vi "test-pose2d.vi"(8 "error in (no error)":errorcluster) -> (0 "error out":errorcluster, 3 "All PASSED":bool)   [LabVIEW 2019]
uses:
  <vilib>/Rock Robotics/WPI/ThirdParty/JAS_Junk/TrajLib/Translation_Equals.vi
  <vilib>/Rock Robotics/WPI/ThirdParty/JAS_Junk/TrajLib/Rotation_Equals.vi
  <vilib>/Rock Robotics/WPI/ThirdParty/JAS_Junk/TrajLib/Transform_Create_PosePose.vi
  <vilib>/Rock Robotics/WPI/ThirdParty/JAS_Junk/TrajLib/Pose_TransformBy.vi
  <vilib>/Rock Robotics/WPI/ThirdParty/JAS_Junk/TrajLib/Util_CalcDist.vi
  <vilib>/Rock Robotics/WPI/ThirdParty/JAS_Junk/TrajLib/Rotation_UnaryMinus.vi
  <vilib>/Rock Robotics/WPI/ThirdParty/JAS_Junk/TrajLib/Translation_RotateBy.vi
  <vilib>/Rock Robotics/WPI/ThirdParty/JAS_Junk/TrajLib/Translation_Minus.vi
  <vilib>/Rock Robotics/WPI/ThirdParty/JAS_Junk/TrajLib/Rotation_Minus.vi
  <vilib>/Rock Robotics/WPI/ThirdParty/JAS_Junk/TrajLib/Translation_Plus.vi
  <vilib>/Rock Robotics/WPI/ThirdParty/JAS_Junk/TrajLib/Rotation_Plus.vi
  <vilib>/Rock Robotics/WPI/ThirdParty/JAS_Junk/TrajLib/Rotation_RotateBy.vi
  <vilib>/Rock Robotics/WPI/ThirdParty/JAS_Junk/TrajLib/Rotation_CreateXY.vi
  <vilib>/Rock Robotics/WPI/ThirdParty/JAS_Junk/TrajLib/Trajectory_Library.lvlib
panel:
  out "T4 -- Deg -- 0":dbl
  out "T4 -- y -- 0":dbl
  out "T4 -- X -- 0":dbl
  out "T3 - False":bool
  out "T2 - True":bool
  out "T1 -- Deg -- 0":dbl
  out "T1 -- y -- 0":dbl
  out "T1 -- X -- 0":dbl
  out "T0 -- Deg -- 0":dbl
  out "T0 -- y -- 0":dbl
  out "T0 -- X -- 0":dbl
  # "Pose 2D test"
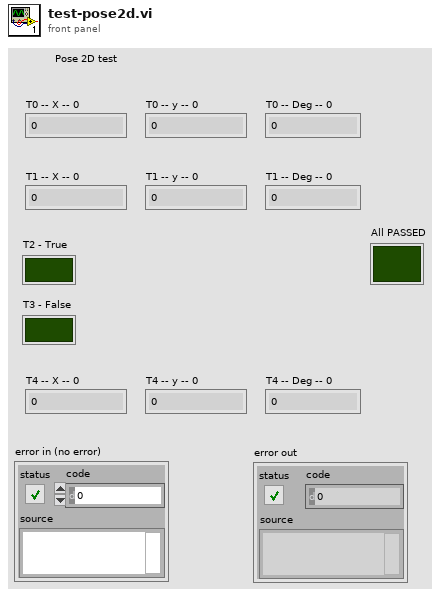
[diagram p1: front panel]
types:
  T1 = typedef "Trajectory_Library.lvlib/TRANSLATION2D.ctl" = cluster{"X":dbl, "Y":dbl}
  T2 = typedef "Trajectory_Library.lvlib/ROTATION2D.ctl" = cluster{"VALUE":dbl, "COS":dbl, "SIN":dbl}
  T3 = typedef "Trajectory_Library.lvlib/TRANSFORM2D.ctl" = cluster{"TRANSLATION":T1, "ROTATION":T2}
  T4 = typedef "Trajectory_Library.lvlib/POSE2D.ctl" = cluster{"TRANSLATION":T1, "ROTATION":T2}
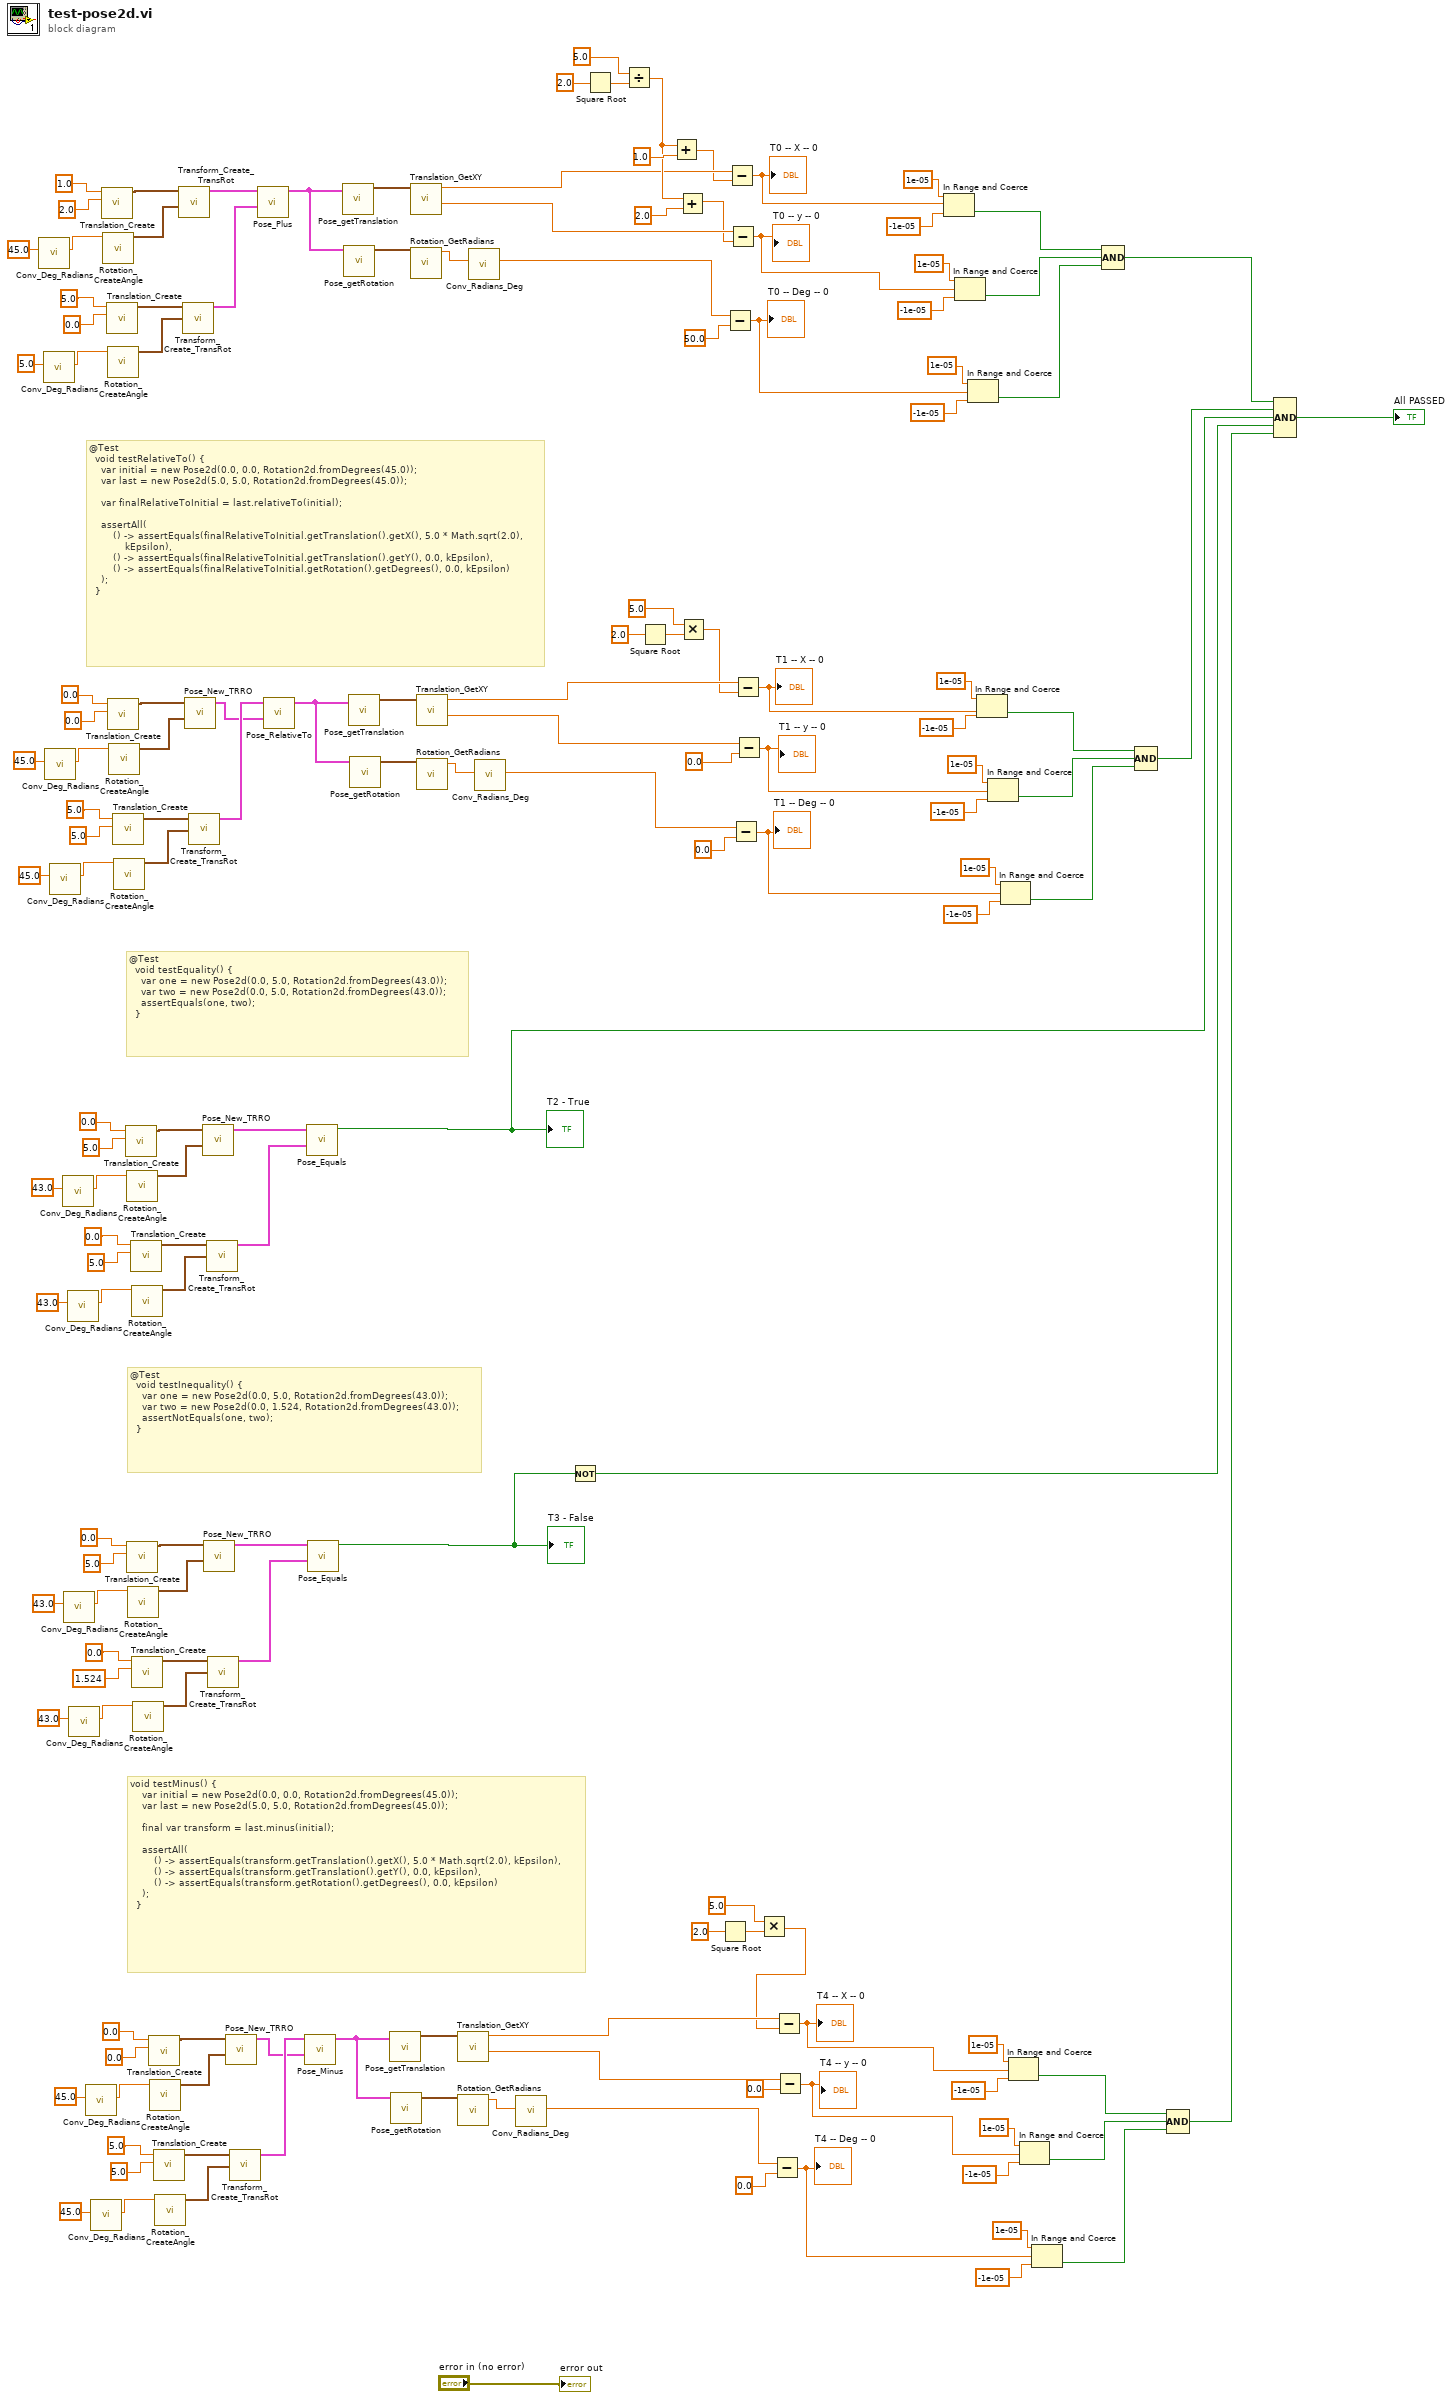
[diagram p0: block diagram]
diagram:
  # "void testMinus() {\n    var initial = new Pose2d(0.0, 0.0, Rotation2d.fromDegrees(45.0));\n    var last = new Pose2d(5.0, 5.0, Rotation2d.fromDegrees(45.0));\n\n    final var transform = last.minus(initial);\n\n    assertAll(\n        () -> assertEquals(transform.getTranslation().getX(), 5.0 * Math.sqrt(2.0), kEpsilon),\n        () -> assertEquals(transform.getTranslation().getY(), 0.0, kEpsilon),\n        () -> assertEquals(transform.getRotation().getDegrees(), 0.0, kEpsilon)\n    );\n  }"
  # "@Test\n  void testInequality() {\n    var one = new Pose2d(0.0, 5.0, Rotation2d.fromDegrees(43.0));\n    var two = new Pose2d(0.0, 1.524, Rotation2d.fromDegrees(43.0));\n    assertNotEquals(one, two);\n  }"
  # "@Test\n  void testEquality() {\n    var one = new Pose2d(0.0, 5.0, Rotation2d.fromDegrees(43.0));\n    var two = new Pose2d(0.0, 5.0, Rotation2d.fromDegrees(43.0));\n    assertEquals(one, two);\n  }"
  # "@Test\n  void testRelativeTo() {\n    var initial = new Pose2d(0.0, 0.0, Rotation2d.fromDegrees(45.0));\n    var last = new Pose2d(5.0, 5.0, Rotation2d.fromDegrees(45.0));\n\n    var finalRelativeToInitial = last.relativeTo(initial);\n\n    assertAll(\n        () -> assertEquals(finalRelativeToInitial.getTranslation().getX(), 5.0 * Math.sqrt(2.0),\n            kEpsilon),\n        () -> assertEquals(finalRelativeToInitial.getTranslation().getY(), 0.0, kEpsilon),\n        () -> assertEquals(finalRelativeToInitial.getRotation().getDegrees(), 0.0, kEpsilon)\n    );\n  }"
  n1 = call <vilib>:"Conv_Deg_Radians.vi"("Degress"=45.0) -> ("Radians"=w153:dbl)  [unwired: 10 in]
  n2 = call <vilib>:"Conv_Deg_Radians.vi"("Degress"=5.0) -> ("Radians"=w148:dbl)  [unwired: 10 in]
  n3 = call <vilib>:"Conv_Deg_Radians.vi"("Degress"=45.0) -> ("Radians"=w123:dbl)  [unwired: 10 in]
  n4 = call <vilib>:"Conv_Deg_Radians.vi"("Degress"=45.0) -> ("Radians"=w118:dbl)  [unwired: 10 in]
  n5 = call <vilib>:"Conv_Deg_Radians.vi"("Degress"=43.0) -> ("Radians"=w96:dbl)  [unwired: 10 in]
  n6 = call <vilib>:"Conv_Deg_Radians.vi"("Degress"=43.0) -> ("Radians"=w82:dbl)  [unwired: 10 in]
  n7 = call <vilib>:"Conv_Deg_Radians.vi"("Degress"=43.0) -> ("Radians"=w91:dbl)  [unwired: 10 in]
  n8 = call <vilib>:"Conv_Deg_Radians.vi"("Degress"=43.0) -> ("Radians"=w77:dbl)  [unwired: 10 in]
  n9 = call <vilib>:"Conv_Deg_Radians.vi"("Degress"=45.0) -> ("Radians"=w68:dbl)  [unwired: 10 in]
  n10 = call <vilib>:"Conv_Deg_Radians.vi"("Degress"=45.0) -> ("Radians"=w63:dbl)  [unwired: 10 in]
  n11 = call <vilib>:"Translation_Create.vi"("Y"=2.0, "X"=1.0) -> ("TRANSLATION"=w152:T1)  [unwired: 9 in]
  n12 = call <vilib>:"Rotation_CreateAngle.vi"("Angle"=w153) -> ("ROTATION"=w151:T2)  [unwired: 10 in]
  n13 = call <vilib>:"Translation_Create.vi"("Y"=0.0, "X"=5.0) -> ("TRANSLATION"=w146:T1)  [unwired: 9 in]
  n14 = call <vilib>:"Rotation_CreateAngle.vi"("Angle"=w148) -> ("ROTATION"=w145:T2)  [unwired: 10 in]
  n15 = call <vilib>:"Translation_Create.vi"("Y"=0.0, "X"=0.0) -> ("TRANSLATION"=w122:T1)  [unwired: 9 in]
  n16 = call <vilib>:"Rotation_CreateAngle.vi"("Angle"=w123) -> ("ROTATION"=w121:T2)  [unwired: 10 in]
  n17 = call <vilib>:"Translation_Create.vi"("Y"=5.0, "X"=5.0) -> ("TRANSLATION"=w116:T1)  [unwired: 9 in]
  n18 = call <vilib>:"Rotation_CreateAngle.vi"("Angle"=w118) -> ("ROTATION"=w115:T2)  [unwired: 10 in]
  n19 = call <vilib>:"Translation_Create.vi"("Y"=5.0, "X"=0.0) -> ("TRANSLATION"=w95:T1)  [unwired: 9 in]
  n20 = call <vilib>:"Rotation_CreateAngle.vi"("Angle"=w96) -> ("ROTATION"=w94:T2)  [unwired: 10 in]
  n21 = call <vilib>:"Translation_Create.vi"("Y"=5.0, "X"=0.0) -> ("TRANSLATION"=w81:T1)  [unwired: 9 in]
  n22 = call <vilib>:"Rotation_CreateAngle.vi"("Angle"=w82) -> ("ROTATION"=w80:T2)  [unwired: 10 in]
  n23 = call <vilib>:"Translation_Create.vi"("Y"=5.0, "X"=0.0) -> ("TRANSLATION"=w89:T1)  [unwired: 9 in]
  n24 = call <vilib>:"Rotation_CreateAngle.vi"("Angle"=w91) -> ("ROTATION"=w88:T2)  [unwired: 10 in]
  n25 = call <vilib>:"Translation_Create.vi"("Y"=1.524, "X"=0.0) -> ("TRANSLATION"=w75:T1)  [unwired: 9 in]
  n26 = call <vilib>:"Rotation_CreateAngle.vi"("Angle"=w77) -> ("ROTATION"=w74:T2)  [unwired: 10 in]
  n27 = call <vilib>:"Translation_Create.vi"("Y"=0.0, "X"=0.0) -> ("TRANSLATION"=w67:T1)  [unwired: 9 in]
  n28 = call <vilib>:"Rotation_CreateAngle.vi"("Angle"=w68) -> ("ROTATION"=w66:T2)  [unwired: 10 in]
  n29 = call <vilib>:"Translation_Create.vi"("Y"=5.0, "X"=5.0) -> ("TRANSLATION"=w61:T1)  [unwired: 9 in]
  n30 = call <vilib>:"Rotation_CreateAngle.vi"("Angle"=w63) -> ("ROTATION"=w60:T2)  [unwired: 10 in]
  n31 = call <vilib>:"Transform_Create_TransRot.vi"("ROTATION"=w151, "TRANSLATION"=w152) -> ("TRANSFORM"=w144:T3)  [unwired: 9 in]
  n32 = call <vilib>:"Transform_Create_TransRot.vi"("ROTATION"=w145, "TRANSLATION"=w146) -> ("TRANSFORM"=w143:T3)  [unwired: 9 in]
  n33 = call <vilib>:"Pose_New_TRRO.vi"("ROTATION"=w121, "TRANSLATION"=w122) -> ("outPOSE"=w101:T4)  [unwired: 9 in]
  n34 = call <vilib>:"Transform_Create_TransRot.vi"("ROTATION"=w115, "TRANSLATION"=w116) -> ("TRANSFORM"=w102:T3)  [unwired: 9 in]
  n35 = call <vilib>:"Pose_New_TRRO.vi"("ROTATION"=w94, "TRANSLATION"=w95) -> ("outPOSE"=w87:T4)  [unwired: 9 in]
  n36 = call <vilib>:"Pose_New_TRRO.vi"("ROTATION"=w80, "TRANSLATION"=w81) -> ("outPOSE"=w73:T4)  [unwired: 9 in]
  n37 = call <vilib>:"Transform_Create_TransRot.vi"("ROTATION"=w88, "TRANSLATION"=w89) -> ("TRANSFORM"=w86:T3)  [unwired: 9 in]
  n38 = call <vilib>:"Transform_Create_TransRot.vi"("ROTATION"=w74, "TRANSLATION"=w75) -> ("TRANSFORM"=w72:T3)  [unwired: 9 in]
  n39 = call <vilib>:"Pose_New_TRRO.vi"("ROTATION"=w66, "TRANSLATION"=w67) -> ("outPOSE"=w47:T4)  [unwired: 9 in]
  n40 = call <vilib>:"Transform_Create_TransRot.vi"("ROTATION"=w60, "TRANSLATION"=w61) -> ("TRANSFORM"=w48:T3)  [unwired: 9 in]
  n41 = call <vilib>:"Pose_Plus.vi"("other TRANSFORM"=w143, "in POSE"=w144) -> ("out POSE"=w141:T4)  [unwired: 9 in]
  n42 = call <vilib>:"Pose_RelativeTo.vi"("other POSE"=w101, "in POSE"=w102) -> ("out POSE"=w113:T4)  [unwired: 9 in]
  n43 = call <vilib>:"Pose_Minus.vi"("other TRANSFORM"=w47, "in POSE"=w48) -> ("outTRANSFORM"=w58:T3)  [unwired: 9 in]
  n44 = call <vilib>:"Pose_Equals.vi"("other POSE"=w86, "in POSE"=w87) -> ("Equals"=w17:bool)  [unwired: 9 in]
  "T2 - True" <- w17
  n45 = call <vilib>:"Pose_Equals.vi"("other POSE"=w72, "in POSE"=w73) -> ("Equals"=w16:bool)  [unwired: 9 in]
  "T3 - False" <- w16
  n46 = call <vilib>:"Pose_getTranslation.vi"("in POSE"=w141) -> ("outTRANSLATION"=w142:T1)  [unwired: 10 in]
  n47 = call <vilib>:"Pose_getRotation.vi"("in POSE"=w141) -> ("out ROTATION"=w140:T2)  [unwired: 10 in]
  n48 = call <vilib>:"Pose_getTranslation.vi"("in POSE"=w113) -> ("outTRANSLATION"=w114:T1)  [unwired: 10 in]
  n49 = call <vilib>:"Pose_getRotation.vi"("in POSE"=w113) -> ("out ROTATION"=w112:T2)  [unwired: 10 in]
  n50 = call <vilib>:"Pose_getTranslation.vi"("in POSE"=w58) -> ("outTRANSLATION"=w59:T1)  [unwired: 10 in]
  n51 = call <vilib>:"Pose_getRotation.vi"("in POSE"=w58) -> ("out ROTATION"=w57:T2)  [unwired: 10 in]
  n52 = call <vilib>:"Translation_GetXY.vi"("In Translation"=w142) -> ("Y"=w131:dbl, "X"=w132:dbl)  [unwired: 9 in]
  n53 = call <vilib>:"Rotation_GetRadians.vi"("in ROTATION"=w140) -> ("AngleRadians"=w139:dbl)  [unwired: 10 in]
  n54 = call <vilib>:"Translation_GetXY.vi"("In Translation"=w114) -> ("Y"=w106:dbl, "X"=w107:dbl)  [unwired: 9 in]
  n55 = call <vilib>:"Rotation_GetRadians.vi"("in ROTATION"=w112) -> ("AngleRadians"=w111:dbl)  [unwired: 10 in]
  n56 = call <vilib>:"Translation_GetXY.vi"("In Translation"=w59) -> ("Y"=w51:dbl, "X"=w52:dbl)  [unwired: 9 in]
  n57 = call <vilib>:"Rotation_GetRadians.vi"("in ROTATION"=w57) -> ("AngleRadians"=w56:dbl)  [unwired: 10 in]
  n58 = call <vilib>:"Conv_Radians_Deg.vi"("Radians"=w139) -> ("Degrees"=w127:dbl)  [unwired: 10 in]
  n59 = call <vilib>:"Conv_Radians_Deg.vi"("Radians"=w111) -> ("Degrees"=w104:dbl)  [unwired: 10 in]
  n60 = call <vilib>:"Conv_Radians_Deg.vi"("Radians"=w56) -> ("Degrees"=w49:dbl)  [unwired: 10 in]
  n61 = Not(x=w16) -> (.not. x?=w15:bool)
  n62 = Square Root(x=2.0) -> (sqrt(x)=w137:dbl)
  n63 = Divide(x=5.0, y=w137) -> (x/y=w133:dbl)
  n64 = Square Root(x=2.0) -> (sqrt(x)=w109:dbl)
  n65 = Add(x=w133, y=1.0) -> (x+y=w129:dbl)
  n66 = Add(x=w133, y=2.0) -> (x+y=w130:dbl)
  n67 = Multiply(x=5.0, y=w109) -> (x*y=w100:dbl)
  n68 = Square Root(x=2.0) -> (sqrt(x)=w54:dbl)
  n69 = Subtract(x=w127, y=50.0) -> (x-y=w36:dbl)
  "T0 -- Deg -- 0" <- w36
  n70 = Subtract(x=w132, y=w129) -> (x-y=w38:dbl)
  "T0 -- X -- 0" <- w38
  n71 = Subtract(x=w131, y=w130) -> (x-y=w37:dbl)
  "T0 -- y -- 0" <- w37
  n72 = Subtract(x=w104, y=0.0) -> (x-y=w19:dbl)
  "T1 -- Deg -- 0" <- w19
  n73 = Subtract(x=w107, y=w100) -> (x-y=w21:dbl)
  "T1 -- X -- 0" <- w21
  n74 = Subtract(x=w106, y=0.0) -> (x-y=w20:dbl)
  "T1 -- y -- 0" <- w20
  n75 = Multiply(x=5.0, y=w54) -> (x*y=w46:dbl)
  n76 = Subtract(x=w49, y=0.0) -> (x-y=w3:dbl)
  "T4 -- Deg -- 0" <- w3
  n77 = Subtract(x=w52, y=w46) -> (x-y=w5:dbl)
  "T4 -- X -- 0" <- w5
  n78 = Subtract(x=w51, y=0.0) -> (x-y=w4:dbl)
  "T4 -- y -- 0" <- w4
  n79 = In Range and Coerce(upper limit=1e-05, x=w38, lower limit=-1e-05) -> (In Range?=w35:bool)  [unwired: 1 out]
  n80 = In Range and Coerce(upper limit=1e-05, x=w37, lower limit=-1e-05) -> (In Range?=w34:bool)  [unwired: 1 out]
  n81 = In Range and Coerce(upper limit=1e-05, x=w36, lower limit=-1e-05) -> (In Range?=w33:bool)  [unwired: 1 out]
  n82 = In Range and Coerce(upper limit=1e-05, x=w21, lower limit=-1e-05) -> (In Range?=w24:bool)  [unwired: 1 out]
  n83 = In Range and Coerce(upper limit=1e-05, x=w20, lower limit=-1e-05) -> (In Range?=w23:bool)  [unwired: 1 out]
  n84 = In Range and Coerce(upper limit=1e-05, x=w19, lower limit=-1e-05) -> (In Range?=w22:bool)  [unwired: 1 out]
  n85 = In Range and Coerce(upper limit=1e-05, x=w5, lower limit=-1e-05) -> (In Range?=w8:bool)  [unwired: 1 out]
  n86 = In Range and Coerce(upper limit=1e-05, x=w4, lower limit=-1e-05) -> (In Range?=w7:bool)  [unwired: 1 out]
  n87 = In Range and Coerce(upper limit=1e-05, x=w3, lower limit=-1e-05) -> (In Range?=w6:bool)  [unwired: 1 out]
  n88 = Compound Arithmetic op=AND(w35, w34, w33) -> (w32:bool)
  n89 = Compound Arithmetic op=AND(w24, w23, w22) -> (w18:bool)
  n90 = Compound Arithmetic op=AND(w8, w7, w6) -> (w2:bool)
  n91 = Compound Arithmetic op=AND(w32, w18, w17, w15, w2) -> (→"All PASSED":bool)
  "error out" <- "error in (no error)"
